vi "onListenForNewConnection.vi"(8 "error in (no error)":errorcluster, 9 "timeout (ms)":i32=1, 11 "Listener":refnum<class "TCPConnection.lvclass">) -> (0 "error out":errorcluster, 1 "New connection":bool, 3 "New Connection":refnum<class "Connection.lvclass">)   [LabVIEW 2013, in "MQTT_TCP.lvlib" / "TCPConnection.lvclass"]
uses:
  TCPConnection.lvclass
  MQTT_Connection/Connection/Connection.lvclass
  TCPConnection.lvclass/TCPConnection.ctl
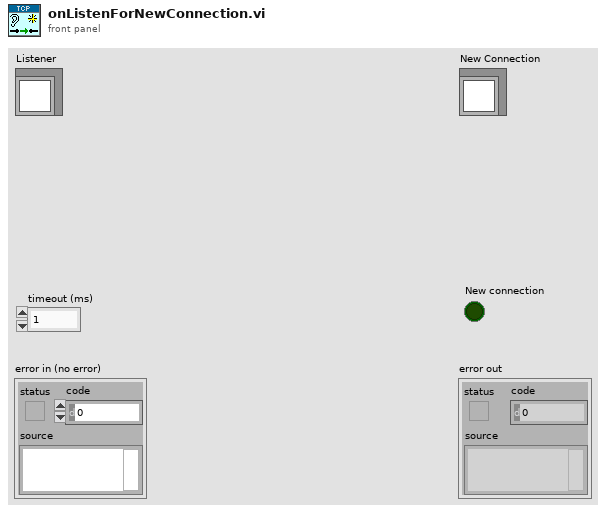
[diagram p1: front panel]
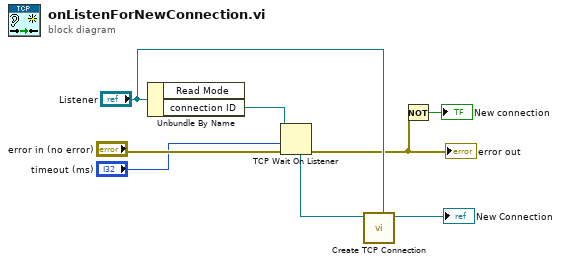
[diagram p0: block diagram]
diagram:
  n1 = Unbundle By Name("Listener") -> ("connection ID"=w6:refnum<k5>)  [unwired: 1 out]
  n2 = TCP Wait On Listener(8:"error in (no error)", 9:"timeout (ms)", 11:w6) -> (0:w1:errorcluster, 4:w4:refnum<k5>)  [unwired: 1 in, 3 out]
  "error out" <- w1
  n3 = call "Create TCP Connection.vi"("TCPConnection in"="Listener", "connection ID"=w4) -> ("TCPConnection out"=→"New Connection":refnum<class "TCPConnection.lvclass">)  [unwired: 8 in, 1 out]
  n4 = Not(x=w1) -> (.not. x?=→"New connection":bool)
